vi "Init Circle.vi"(7 "Color (RGB black)":refnum<class "Color.lvclass">=refnum, 8 "error in (no error)":errorcluster, 9 "diameter (0)":i16, 10 "top left (0,0)":cluster{"x":i16, "y":i16}, 11 "Circle in":refnum<class "Circle.lvclass">) -> (0 "error out":errorcluster, 3 "Circle out":refnum<class "Circle.lvclass">)   [LabVIEW 2020, in "Circle.lvclass"]
doc: "Initialize a circle"
uses:
  Circle.lvclass
  D:/Git/Labview-Libraries/Tools/Drawing Tool Folder/Ellipse/Ellipse.lvclass
  Color/Color.lvclass
  RGB Color/RGB Color.lvclass
  Circle.lvclass/Circle.ctl
  Ellipse/Ellipse.lvclass
panel:
  # "expressionflow.com"
  # "Copyright (c) 2008 Tomi Maila. All rights reserved."
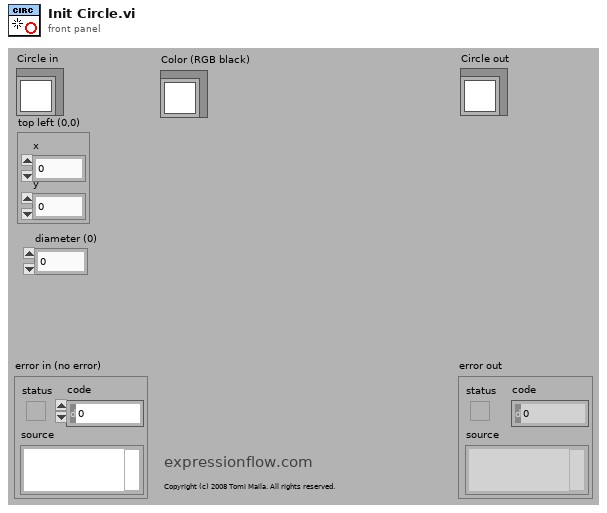
[diagram p1: front panel]
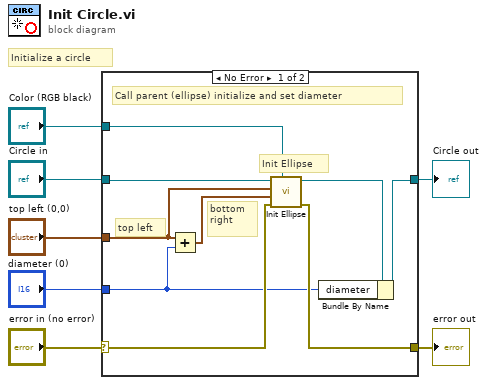
[diagram p0: block diagram]
diagram:
  # "Initialize a circle"
  n1 = case shown="No Error" "error in (no error)" {
    selector: "error in (no error)" -> [w13 w18]
    tunnel: [w14 w18] -> w6
    tunnel: [w10 w17] -> w4
    tunnel: "Circle in" -> [w16 w17]
    tunnel: "top left (0,0)" -> [w12 _]
    tunnel: "diameter (0)" -> [w9 _]
    tunnel: "Color (RGB black)" -> [w15 _]
    frame No Error {
      # "Init Ellipse"
      # "top left"
      # "bottom\nright"
      # "Call parent (ellipse) initialize and set diameter"
      n2 = Add(x=w12, y=w9) -> (x+y=w8:cluster{"x":i16, "y":i16})
      n3 = call "Init Ellipse.vi"("Color (RGB black)"=w15, "error in (no error)"=w13, "bottom right (0,0)"=w8, "top left (0,0)"=w12, "Ellipse in"=w16) -> ("error out"=w14:errorcluster, "Ellipse out"=w11:refnum<class "Circle.lvclass">)  [unwired: 5 in]
      n4 = Bundle By Name(cluster=w11, "diameter"=w9) -> (w10:refnum<class "Circle.lvclass">)
    }
    frame Error {
    }
  }
  "error out" <- w6
  "Circle out" <- w4
